vi "TowerLight_Init.vi"(0 "object in":refnum<class "TowerLight.lvclass">, 2 "TowerLightRef":refnum<vi>, 5 "error in (no error)":errorcluster) -> (14 "object out":refnum<class "TowerLight.lvclass">, 19 "error out":errorcluster)   [LabVIEW 2014, in "TowerLight.lvclass"]
uses:
  TowerLight.lvclass
  TrafficLight.ctl
  TowerLight.lvclass/TowerLight.ctl
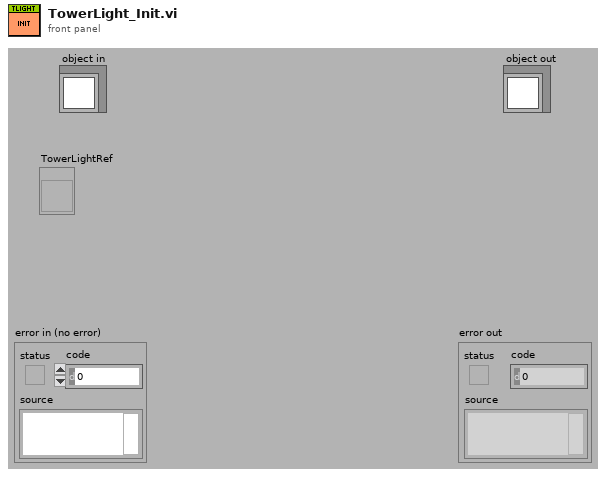
[diagram p1: front panel]
types:
  T1 = typedef "TowerLight.lvclass/TrafficLight.ctl" = cluster{"Red":bool, "Yellow":bool, "Green":bool}
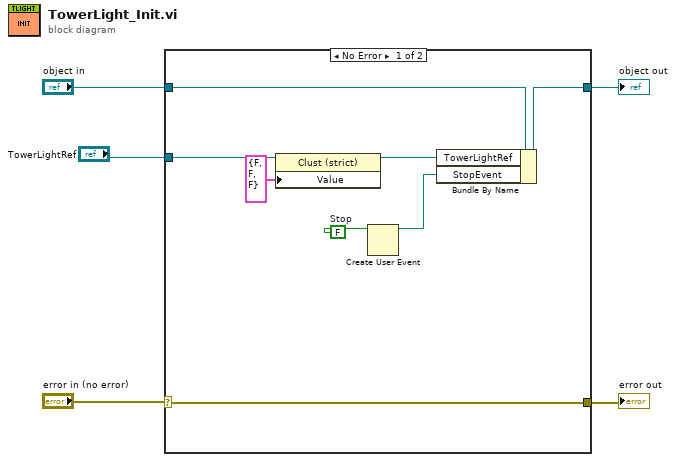
[diagram p0: block diagram]
diagram:
  n1 = case shown="No Error" "error in (no error)" {
    selector: "error in (no error)" -> [w11 w14]
    tunnel: "object in" -> [w13 w15]
    tunnel: [w12 w15] -> w4
    tunnel: [w11 w14] -> w2
    tunnel: "TowerLightRef" -> [w8 _]
    frame No Error {
      w10 = FALSE  # Stop
      n2 = property class="Clust (strict)"(reference=w8, "Value"=T1 {"Red"=FALSE, "Yellow"=FALSE, "Green"=FALSE}) -> (reference out=w7:refnum<vi>)  [unwired: 1 in, 1 out]
      n3 = Create User Event(user event datatype=w10) -> (user event=w9:refnum<user-event>)  [unwired: 1 in, 1 out]
      n4 = Bundle By Name(cluster=w13, "TowerLightRef"=w7, "StopEvent"=w9) -> (w12:refnum<class "TowerLight.lvclass">)
    }
    frame Error {
    }
  }
  "object out" <- w4
  "error out" <- w2
